vi "ImpulseAnalysis.vi"() -> ()   [LabVIEW 2014]
doc: "1. As pulse width increases, the peaks of the spectral analysis narrows and one peak becomes prominent.\n2. Below a certain frequency, the aquisition rate is lower than the frequency and measures peaks at the wrong points\n3. As the number of samples being averaged increases, the noise is reduced"
uses:
  <vilib>/express/express analysis/Spectral/Block/exnSpectralBlock spectral measurements RMS poly.vi
  <vilib>/express/express analysis/Spectral/Block/exnSpectralBlock spectral measurements RMS DDT.vi
  <vilib>/express/express analysis/Spectral/XNode/ExpressSpectralMeasurementsBlockNode.xnode
panel:
  out "FFT":dynamicdata(graph)=[{"t0"=timestamp(0 s since 1904-01-01), "dt"=0.0005, "Y"=array[1000 elements], "attributes"=variant("NI_ChannelName"=variant(string "FFT - (RMS)"))}]
  out "Waveform Graph":dynamicdata(graph)=[{"t0"=timestamp(3499375505.9776244 s since 1904-01-01), "dt"=1.0, "Y"=array[2000 elements]}]
  in  "error in (no error)":errorcluster
  out "error out":errorcluster
  in  "stop":bool
  in  "Time (s)":dbl=0.2
  in  "Rate":dbl=10000.0
  in  "Averages":dbl=20.0
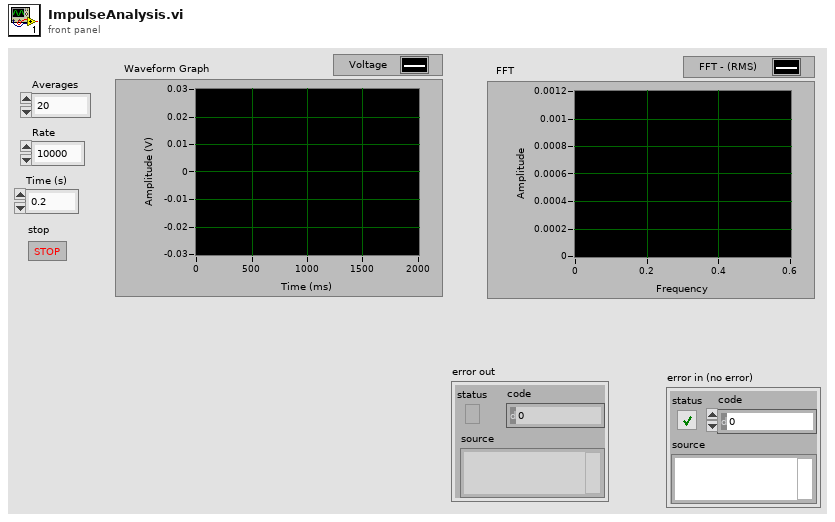
[diagram p1: front panel]
types:
  T1 = cluster{"averaging mode":u16, "weighting mode":u16, "number of averages":u32}
  T2 = cluster{"dB On (F)":bool, "unwrap phase (F)":bool, "convert to degree (F)":bool}
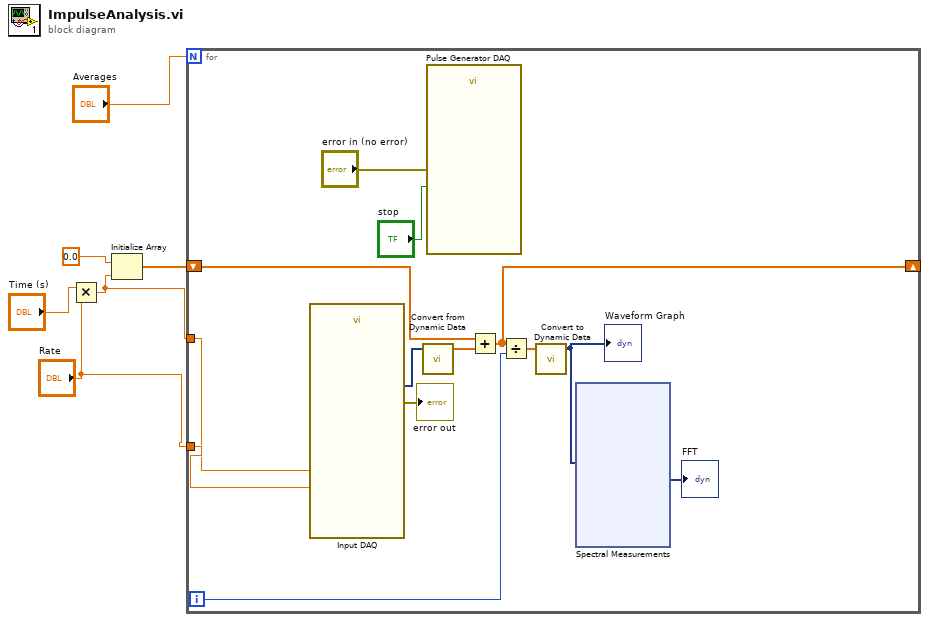
[diagram p0: block diagram]
diagram:
  n1 = Multiply(x="Time (s)", y="Rate") -> (x*y=w1:dbl)
  n2 = Initialize Array(0.0, w1) -> (w5:dbl[])
  n3 = for {
    N: "Averages" -> [_]
    shift-right: [w9] -> _
    shift-left: w5 -> [w13]
    tunnel: "Rate" -> [w15]
    tunnel: w1 -> [w14]
    i -> [w7]
    n4 = call "Input DAQ"("rate"=w15, "number of samples"=w14) -> ("data"=w12:dynamicdata, "error out"=→"error out":errorcluster)  [unwired: 15 in, 1 out]
    n5 = call "Convert from Dynamic Data"("Dynamic Data Type"=w12) -> ("Array"=w11:dbl[])  [unwired: 3 in]
    n6 = call "Pulse Generator DAQ"("error in"="error in (no error)", "stop (T)"="stop") -> ()  [unwired: 16 in, 2 out]
    n7 = Add(x=w13, y=w11) -> (x+y=w9:dbl[])
    n8 = Divide(x=w9, y=w7) -> (x/y=w8:dbl[])
    n9 = call "Convert to Dynamic Data"("Array"=w8) -> ("Dynamic Data Type"=w10:dynamicdata)  [unwired: 3 in]
    "Waveform Graph" <- w10
    n10 = xnode "Spectral Measurements"("Signals"=w10) -> ("FFT - (RMS)"=→"FFT":dynamicdata)  [unwired: 1 in, 2 out]
  }
